vi "H2Purifier_02.vi"() -> ()   [LabVIEW 2011]
panel:
  out "P (Torr)":string
  in  "Prev Button":bool
  out "flow (sccm)":dbl
  in  "Display\nN2     H2":bool
  out "H2 setpoint":string caption="H2 setpoint (sccm)"
  out "N2 setpoint":string caption="N2 setpoint (sccm)"
  out "MANIFOLD N2":bool
  out "MANIFOLD H2":bool
  out "Main message":string
  out "Bleed message":string
  out "UPH message":string
  in  "AdapTorr Close":bool caption="Close"
  out "Close LED":bool caption="Open"
  in  "AdapTorr Open":bool caption="Open"
  out "Open LED":bool caption="Open"
  in  "Vac\nExhuast":bool
  in  "Step":i16
  in  "Next Button":bool caption="OK Button"
  out "Feed":bool
  out "Pump":bool
  out "Purge":bool
  out "Evac":bool
  in  "Tab Control":enum32{"Start up", "Idle"}(tab)
  # "setpoint to ~100 sccm"
  # "sepoint ~200 sccm\nFlow will drop to ~0 sccm"
  # "AdapTorr"
  # "H2 Purifier"
  # "BLEED\nGAS"
  # "UPH FLOW"
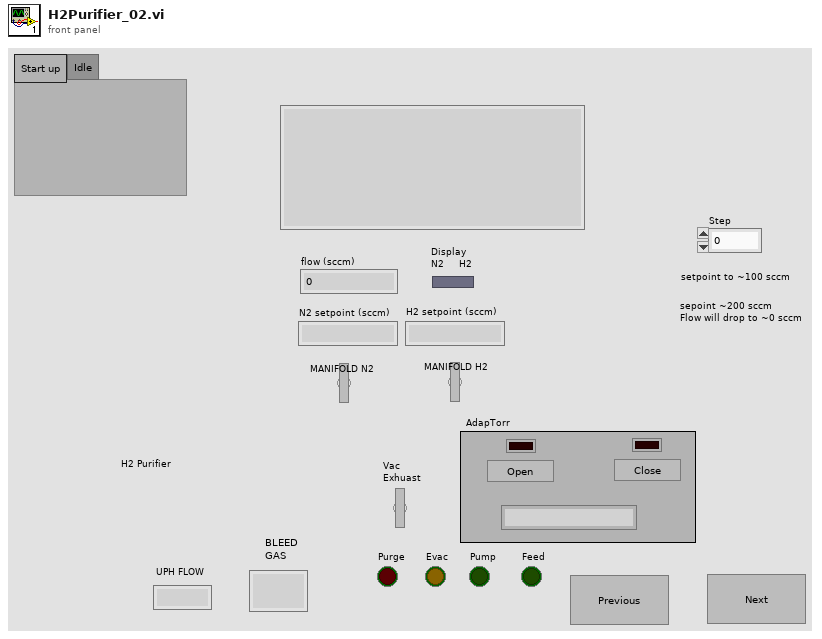
[diagram p1: front panel]
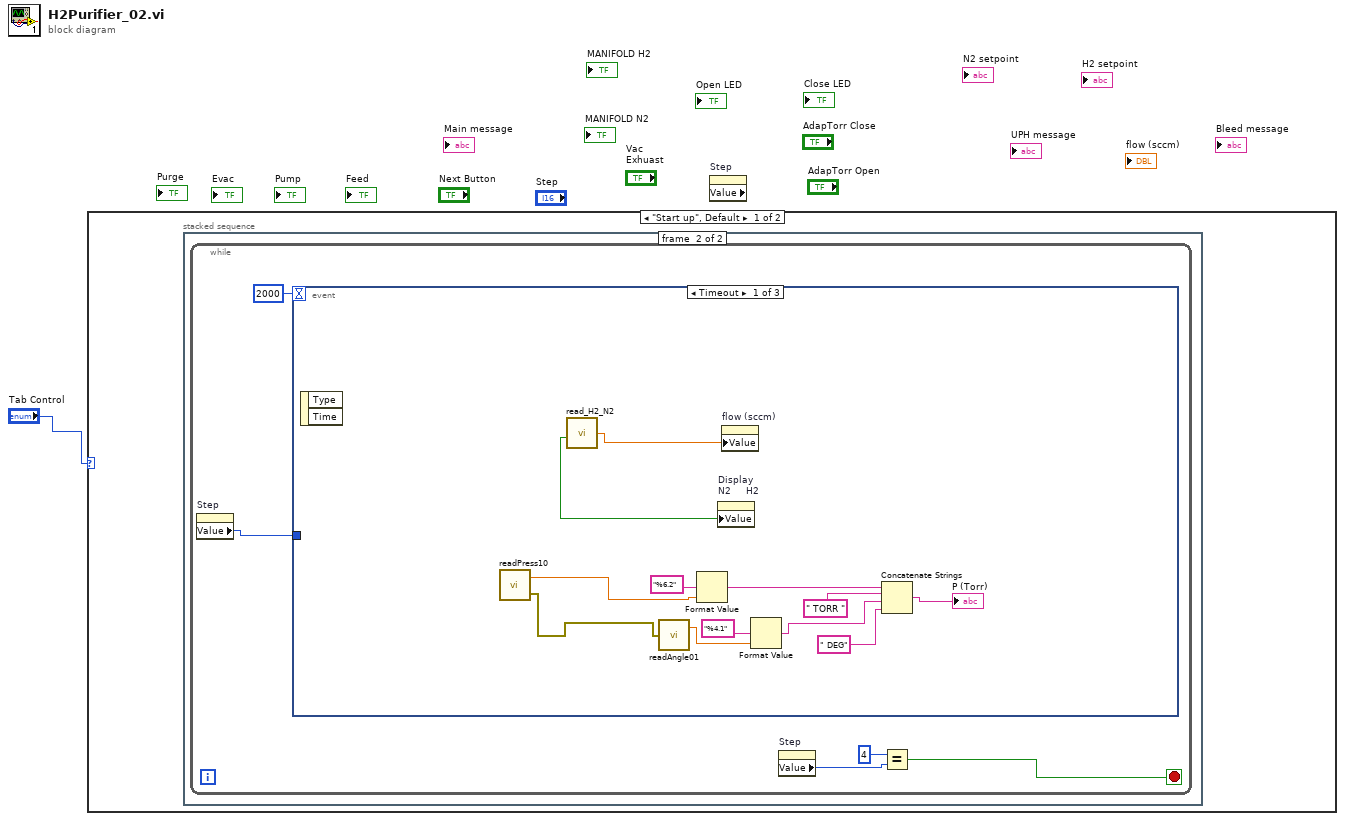
[diagram p0: block diagram]
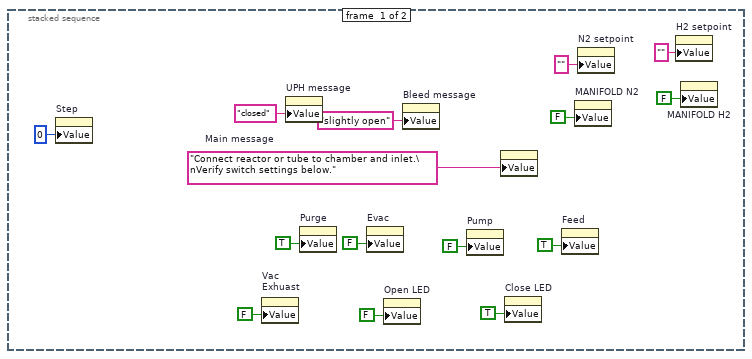
[diagram p2: hidden frame]
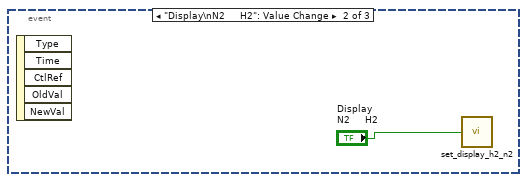
[diagram p3: hidden frame]
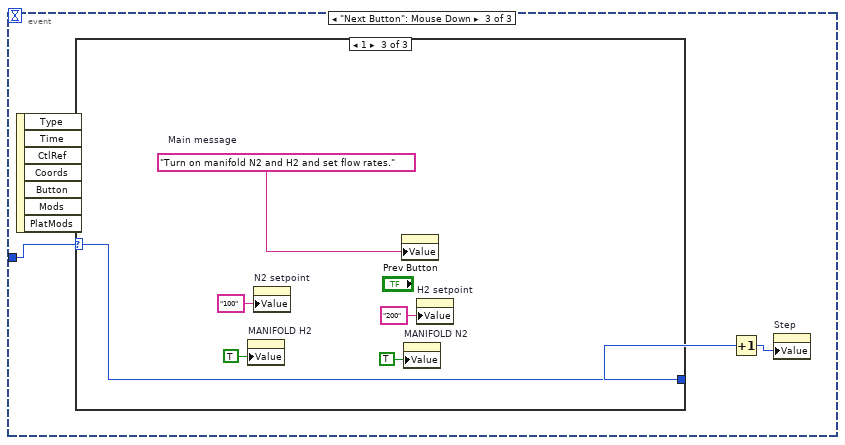
[diagram p4: hidden frame]
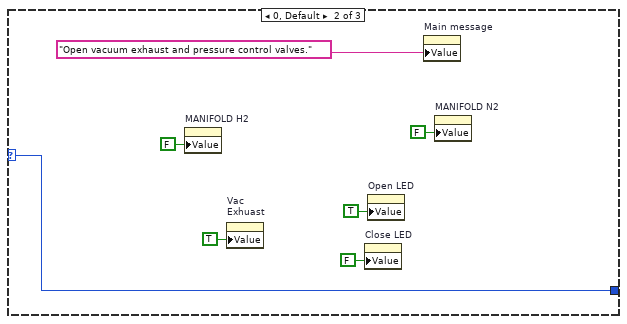
[diagram p6: hidden frame]
diagram:
  n1 = case shown="\"Start up\", Default" "Tab Control" {
    frame "Start up", Default {
      n2 = stacked-sequence {
        frame #0 {
          n3 = property on="Step" class="DigNum (strict)"("Value"=i16 0 ("Step")) -> ()  [unwired: 2 in, 2 out]
          n4 = property on="Vac\nExhuast" class="Bool (strict)"("Value"=FALSE ("Vac\nExhuast")) -> ()  [unwired: 2 in, 2 out]
          n5 = property on="UPH message" class="Str"("Value"="closed" ("UPH message")) -> ()  [unwired: 2 in, 2 out]
          n6 = property on="Purge" class="Bool (strict)"("Value"=TRUE ("Purge")) -> ()  [unwired: 2 in, 2 out]
          n7 = property on="Evac" class="Bool (strict)"("Value"=FALSE ("Evac")) -> ()  [unwired: 2 in, 2 out]
          n8 = property on="Open LED" class="Bool (strict)"("Value"=FALSE ("Open LED")) -> ()  [unwired: 2 in, 2 out]
          n9 = property on="Bleed message" class="Str"("Value"="slightly open" ("Bleed message")) -> ()  [unwired: 2 in, 2 out]
          n10 = property on="Pump" class="Bool (strict)"("Value"=FALSE ("Pump")) -> ()  [unwired: 2 in, 2 out]
          n11 = property on="Main message" class="Str"("Value"="Connect reactor or tube to chamber and inlet.\nVerify switch settings below." ("String")) -> ()  [unwired: 2 in, 2 out]
          n12 = property on="Close LED" class="Bool (strict)"("Value"=TRUE ("Close LED")) -> ()  [unwired: 2 in, 2 out]
          n13 = property on="Feed" class="Bool (strict)"("Value"=TRUE ("Feed")) -> ()  [unwired: 2 in, 2 out]
          n14 = property on="MANIFOLD N2" class="Bool (strict)"("Value"=FALSE ("MANIFOLD N2")) -> ()  [unwired: 2 in, 2 out]
          n15 = property on="N2 setpoint" class="Str"("Value"="" ("N2 setpoint")) -> ()  [unwired: 2 in, 2 out]
          n16 = property on="H2 setpoint" class="Str"("Value"="" ("H2 setpoint")) -> ()  [unwired: 2 in, 2 out]
          n17 = property on="MANIFOLD H2" class="Bool (strict)"("Value"=FALSE ("MANIFOLD H2")) -> ()  [unwired: 2 in, 2 out]
        }
        frame #1 {
          n18 = while {
            stop <- w19 stop-if-true
            n19 = property on="Step" class="DigNum (strict)"() -> ("Value"=w18:i16)  [unwired: 2 in, 2 out]
            n20 = event shown="[0] Timeout" {
              selector: _ -> [_ _ _]
              dyn-events: _ -> [_ _ _]
              timeout: 2000 -> [_ _ _]
              tunnel: w18 -> [_ _ w37]
              event Timeout {
                n21 = event-data() -> ()  [unwired: 1 in, 2 out]
                n22 = call "readPress10.vi"() -> ("P"=w30:dbl, "error out"=w27:errorcluster)  [unwired: 1 in]
                n23 = call "read_H2_N2.vi"() -> ("H2N2 Flow Rate"=w33:dbl, "Display H2N2"=w32:bool)  [unwired: 3 out]
                n24 = call "readAngle01.vi"("error in"=w27) -> ("angle"=w26:dbl)  [unwired: 1 out]
                n25 = Format Value(format string="%6.2", value (0)=w30) -> (output string=w29:string)  [unwired: 1 in]
                n26 = property on="Display\nN2     H2" class="Bool (strict)"("Value"=w32) -> ()  [unwired: 2 in, 2 out]
                n27 = property on="flow (sccm)" class="DigNum (strict)"("Value"=w33) -> ()  [unwired: 2 in, 2 out]
                n28 = Format Value(format string="%4.1", value (0)=w26) -> (output string=w24:string)  [unwired: 1 in]
                n29 = Concatenate Strings(w29, " TORR ", w24, " DEG") -> (→"P (Torr)":string)
              }
              event "Display\nN2     H2": Value Change {
                n30 = event-data() -> ()  [unwired: 1 in, 5 out]
                n31 = call "set_display_h2_n2.vi"("Display H2 or N2"="Display\nN2     H2") -> ()
              }
              event "Next Button": Mouse Down {
                n32 = event-data() -> ()  [unwired: 1 in, 7 out]
                n33 = case shown="1" w37 {
                  selector: w37 -> [w38 w41 w50]
                  tunnel: [w38 w41 w50] -> w35
                  frame 2 {
                  }
                  frame 0, Default {
                    n34 = property on="MANIFOLD H2" class="Bool (strict)"("Value"=FALSE ("MANIFOLD H2")) -> ()  [unwired: 2 in, 2 out]
                    n35 = property on="Vac\nExhuast" class="Bool (strict)"("Value"=TRUE ("Vac\nExhuast")) -> ()  [unwired: 2 in, 2 out]
                    n36 = property on="Close LED" class="Bool (strict)"("Value"=FALSE ("Close LED")) -> ()  [unwired: 2 in, 2 out]
                    n37 = property on="Open LED" class="Bool (strict)"("Value"=TRUE ("Open LED")) -> ()  [unwired: 2 in, 2 out]
                    n38 = property on="Main message" class="Str"("Value"="Open vacuum exhaust and pressure control valves." ("Main message")) -> ()  [unwired: 2 in, 2 out]
                    n39 = property on="MANIFOLD N2" class="Bool (strict)"("Value"=FALSE ("MANIFOLD N2")) -> ()  [unwired: 2 in, 2 out]
                  }
                  frame 1 {
                    n40 = property on="MANIFOLD H2" class="Bool (strict)"("Value"=TRUE ("MANIFOLD H2")) -> ()  [unwired: 2 in, 2 out]
                    n41 = property on="N2 setpoint" class="Str"("Value"="100" ("N2 setpoint")) -> ()  [unwired: 2 in, 2 out]
                    n42 = property on="Main message" class="Str"("Value"="Turn on manifold N2 and H2 and set flow rates." ("String")) -> ()  [unwired: 2 in, 2 out]
                    n43 = property on="MANIFOLD N2" class="Bool (strict)"("Value"=TRUE ("MANIFOLD N2")) -> ()  [unwired: 2 in, 2 out]
                    n44 = property on="H2 setpoint" class="Str"("Value"="200" ("H2 setpoint")) -> ()  [unwired: 2 in, 2 out]
                  }
                }
                n45 = Increment(x=w35) -> (x+1=w36:i16)
                n46 = property on="Step" class="DigNum (strict)"("Value"=w36) -> ()  [unwired: 2 in, 2 out]
              }
            }
            n47 = property on="Step" class="DigNum (strict)"() -> ("Value"=w21:i16)  [unwired: 2 in, 2 out]
            n48 = Equal?(x=i16 4, y=w21) -> (x = y?=w19:bool)
          }
        }
      }
    }
    frame "Idle" {
      n49 = stacked-sequence {
        frame #0 {
        }
      }
    }
  }
  n50 = property on="Step" class="DigNum (strict)" props=["Value"]() -> ()  [unwired: 2 in, 3 out]
